vi "RT Main.vi"() -> ()   [LabVIEW 2022 SP3]
uses:
  RT Controls/RT All Notifer.ctl
  RT Controls/Main RT Case.ctl
  RT Sub VI's/RT Global.vi
panel:
  out "Iteration":i32
  out "Status":bool
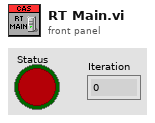
[diagram p1: front panel]
types:
  T1 = enum16{"Init", "Read 'All'", "Read 'n'", "Read '1'", "Write '1'", "Write 'n'", "Write 'All'"}
  T2 = typedef "Main RT Case.ctl" = enum16{"initialize", "Wait For Command", "Wai For Connection"}
  T3 = typedef "RT All Notifer.ctl" = cluster{"Start DAQ":refnum<notifier>, "Sequence":refnum<notifier>}
  T4 = typedef "RT All Queue.ctl" = cluster{"AI\nAO\nDO\nTC\nACC\nStrain":refnum<queue>[], "DI":refnum<queue>}
  T5 = cluster{"Activate Task":cluster{"Analog input":bool, "Analog Output":bool, "Digital input":bool, "Digital output":bool, "Thermocouple":bool, "Strain Gauge":bool, "Accelerometer":bool}, "Start DAQ":bool, "Start Time":timestamp, "DO Names":string[], "AO Names":string[], "AO Default":dbl[], "DO Default":bool[], "Config":cluster{"AO config":cluster{"Channel_Name":string, "Channel_Number":string, "Default_Value":dbl, "Units":string}[], "AI config":cluster{"Channel_Name":string, "Channel_Number":string, "Pre_Scale_min":dbl, "Pre_Scale_max":dbl, "Sensor_min":dbl, "Sensor_max":dbl, "Units":string}[], "DI config":cluster{"Channel_Name":string, "Channel_Number":string, "Default_Value":bool, "DI invert?":bool}[], "DO config":cluster{"Channel_Name":string, "Channel_Number":string, "Default_Value":bool, "DO invert?":bool}[], "TC config":cluster{"Channel_Name":string, "Channel_Number":string, "Pre_Scale_min":dbl, "Pre_Scale_max":dbl, "units":i32, " type":i32}[], "ACC config":cluster{"Channel_Name":string, "Channel_Number":string, "Pre_Scale_min":dbl, "Pre_Scale_max":dbl, "Terminal configuration":i32, "Sensitivity":dbl, "Sensitivity units":i32}[], "SG config":cluster{"Channel_Name":string, "Channel_Number":string, "Pre_Scale_min":dbl, "Pre_Scale_max":dbl}[], "Strain Gauge Settings":cluster{"poisson ratio":dbl, "nominal gage resistance":dbl, "gage factor":dbl}, "Bridge Settings":cluster{"voltage excitation value":dbl, "voltage excitation source":i32, "initial bridge voltage":dbl, "lead wire resistance":dbl, "strain configuration":i32}, "Sample Rate":cluster{"AI Sample Rate":dbl, "AO Sample Rate":dbl, "DI Sample Rate":dbl, "TC Sample Rate":dbl, "DO Sample Rate":dbl, "SG Sample Rate":dbl, "ACC Sample Rate":dbl}}}
  T6 = cluster{"AO":cluster{"CDT":dbl, "Range":dbl, "Component ID":string}[], "DO":cluster{"CDT":dbl, "Position":bool, "Component ID":string}[], "Launch Time":timestamp}
  T7 = cluster{"AO config":cluster{"Channel_Name":string, "Channel_Number":string, "Default_Value":dbl, "Units":string}[], "AI config":cluster{"Channel_Name":string, "Channel_Number":string, "Pre_Scale_min":dbl, "Pre_Scale_max":dbl, "Sensor_min":dbl, "Sensor_max":dbl, "Units":string}[], "DI config":cluster{"Channel_Name":string, "Channel_Number":string, "Default_Value":bool, "DI invert?":bool}[], "DO config":cluster{"Channel_Name":string, "Channel_Number":string, "Default_Value":bool, "DO invert?":bool}[], "TC config":cluster{"Channel_Name":string, "Channel_Number":string, "Pre_Scale_min":dbl, "Pre_Scale_max":dbl, "units":i32, " type":i32}[], "ACC config":cluster{"Channel_Name":string, "Channel_Number":string, "Pre_Scale_min":dbl, "Pre_Scale_max":dbl, "Terminal configuration":i32, "Sensitivity":dbl, "Sensitivity units":i32}[], "SG config":cluster{"Channel_Name":string, "Channel_Number":string, "Pre_Scale_min":dbl, "Pre_Scale_max":dbl}[], "Strain Gauge Settings":cluster{"poisson ratio":dbl, "nominal gage resistance":dbl, "gage factor":dbl}, "Bridge Settings":cluster{"voltage excitation value":dbl, "voltage excitation source":i32, "initial bridge voltage":dbl, "lead wire resistance":dbl, "strain configuration":i32}, "Sample Rate":cluster{"AI Sample Rate":dbl, "AO Sample Rate":dbl, "DI Sample Rate":dbl, "TC Sample Rate":dbl, "DO Sample Rate":dbl, "SG Sample Rate":dbl, "ACC Sample Rate":dbl}}
  T8 = cluster{"Analog input":bool, "Analog Output":bool, "Digital input":bool, "Digital output":bool, "Thermocouple":bool, "Strain Gauge":bool, "Accelerometer":bool}
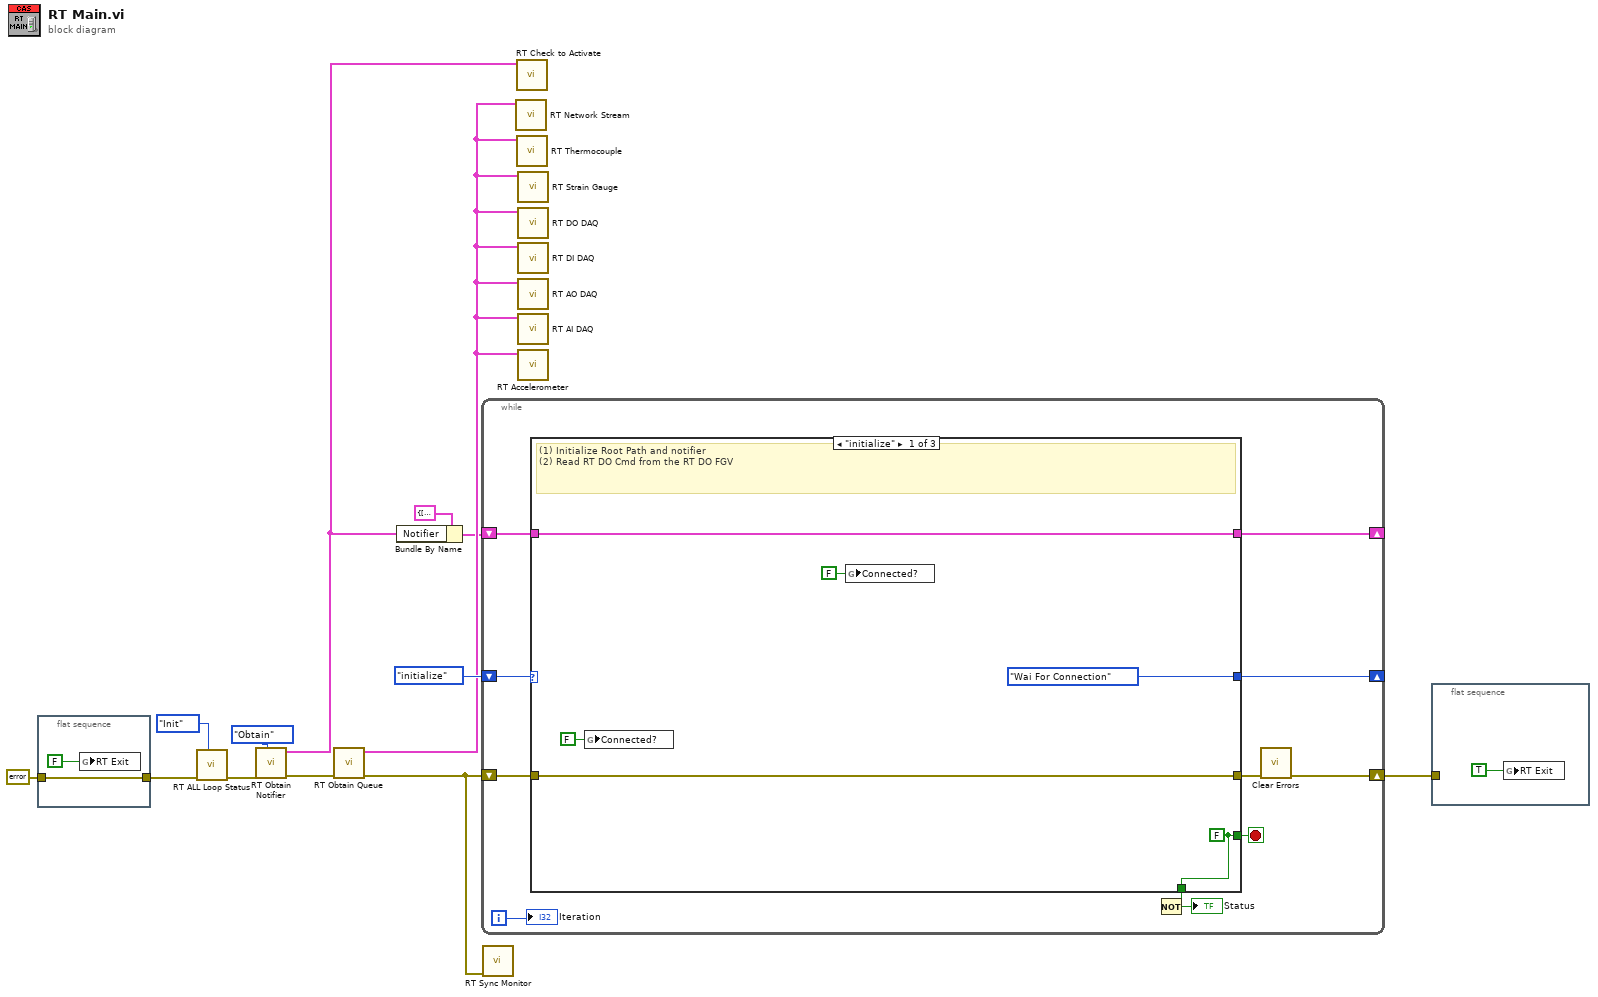
[diagram p0: block diagram]
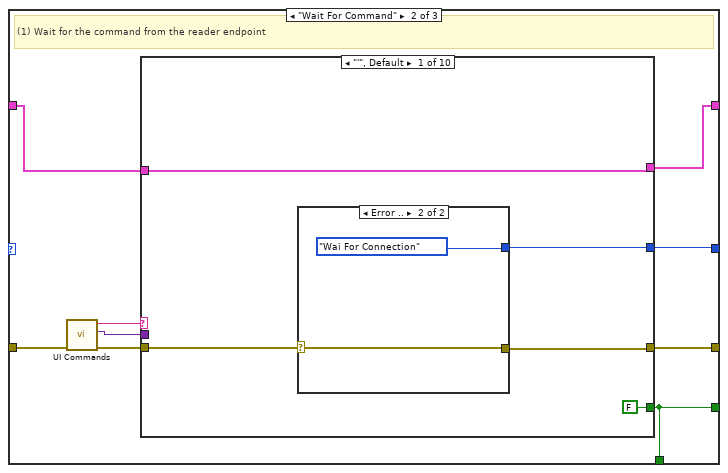
[diagram p2: hidden frame]
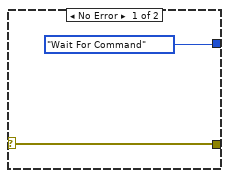
[diagram p3: hidden frame]
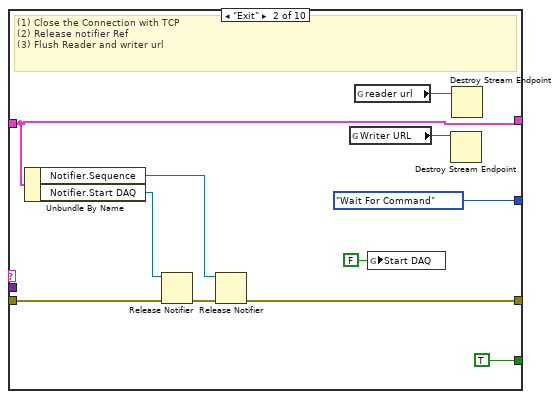
[diagram p4: hidden frame]
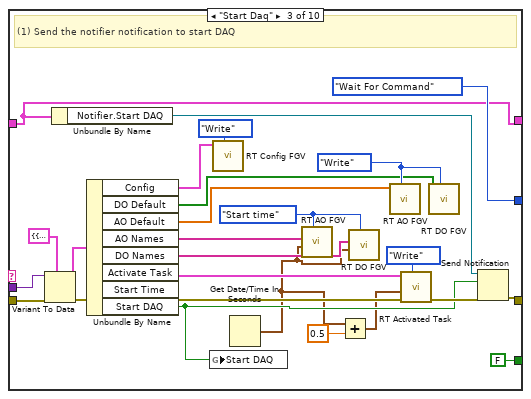
[diagram p5: hidden frame]
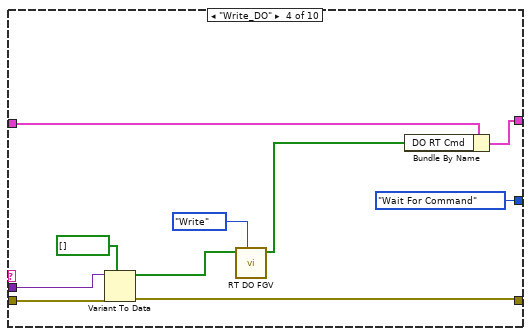
[diagram p6: hidden frame]
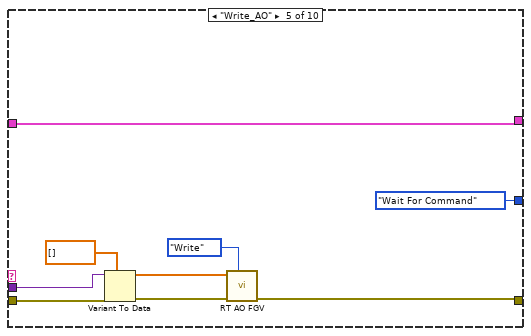
[diagram p7: hidden frame]
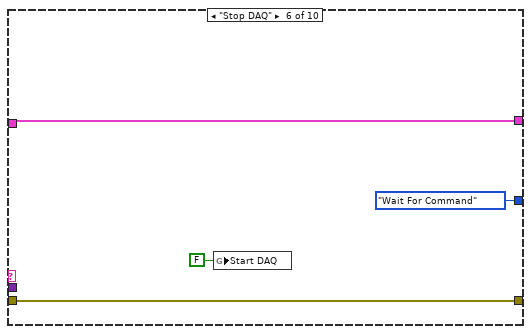
[diagram p8: hidden frame]
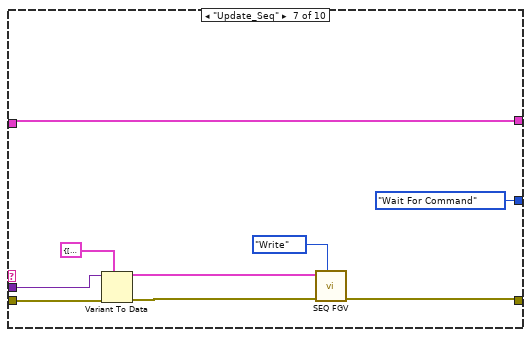
[diagram p9: hidden frame]
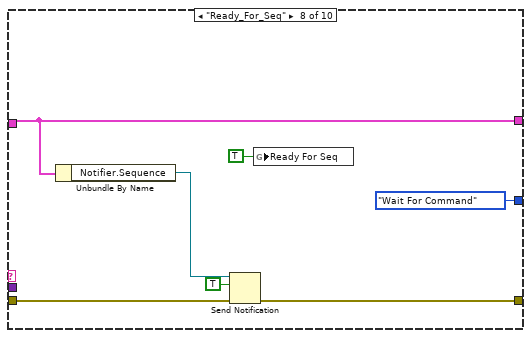
[diagram p10: hidden frame]
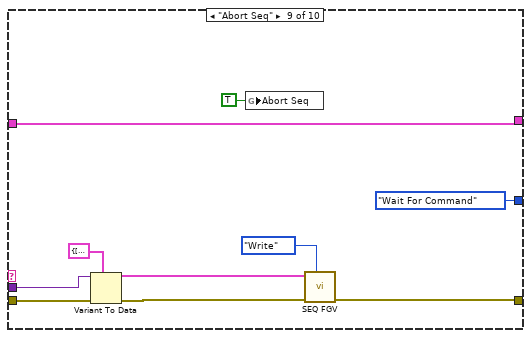
[diagram p11: hidden frame]
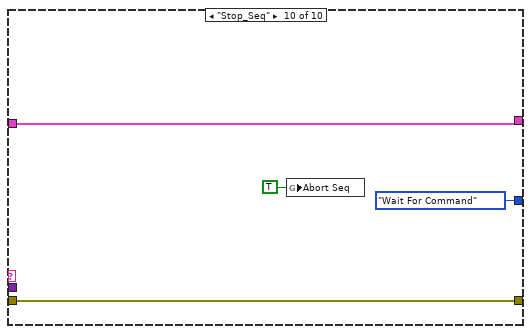
[diagram p12: hidden frame]
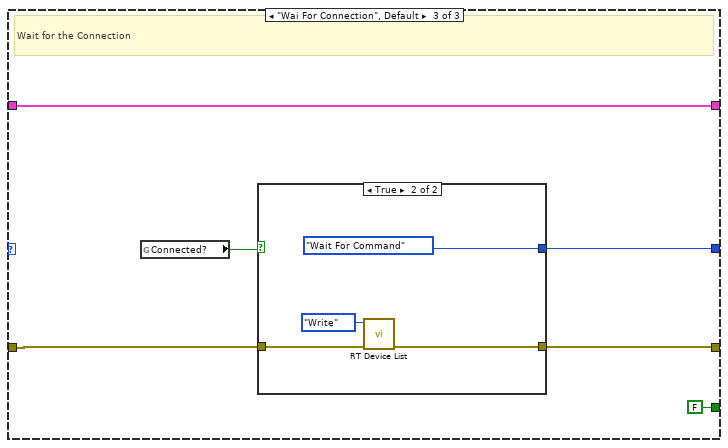
[diagram p13: hidden frame]
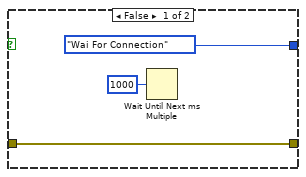
[diagram p14: hidden frame]
diagram:
  n1 = flat-sequence {
    tunnel: errorcluster {"status"=FALSE, "code"=0, "source"=""} ("error in (no error)") -> [w15]
    tunnel: [w15] -> w5
    frame #0 {
      n2 = global write "RT Global.vi" "RT Exit"(FALSE ("Start DAQ")) -> ()
    }
  }
  n3 = call "RT ALL Loop Status.vi"("Option"=T1."Init", "error in (no error)"=w5) -> ("error out"=w4:errorcluster)  [unwired: 7 in, 2 out]
  n4 = call "RT Obtain Notifier.vi"("Case"=enum16{"Obtain", "Read"}."Obtain", "error in (no error)"=w4) -> ("error out"=w8:errorcluster, "All Notifier"=w2:T3)  [unwired: 8 in]
  n5 = call "RT Obtain Queue.vi"("error in"=w8) -> ("error out"=w1:errorcluster, "Queue ref"=w12:T4)  [unwired: 9 in]
  n6 = Bundle By Name(cluster=cluster{"DO RT Cmd":bool[], " Notifier":T3} {"DO RT Cmd"=[], " Notifier"={"Start DAQ"=refnum, "Sequence"=refnum}}, "Notifier"=w2) -> (w6:cluster{"DO RT Cmd":bool[], " Notifier":T3})
  n7 = while {
    shift-right: [w16] -> w11
    shift-left: w1 -> [w25]
    shift-right: [w18] -> _
    shift-left: w6 -> [w17]
    shift-right: [w23] -> _
    shift-left: Main_RT_Case."initialize" -> [w26]
    i -> [w22]
    stop <- w24 stop-if-true
    n8 = case shown="\"initialize\"" w26 {
      tunnel: w25 -> [w32 w36 w140]
      tunnel: [w32 w41 w139] -> w19
      tunnel: [w30 w37 FALSE] -> w24
      tunnel: w17 -> [w31 w40 w144]
      tunnel: [w31 w39 w144] -> w18
      tunnel: [Main_RT_Case."Wai For Connection" w38 w143] -> w23
      tunnel: [w30 w37 _] -> w20
      frame "initialize" {
        w30 = FALSE
        # "(1) Initialize Root Path and notifier\n(2) Read RT DO Cmd from the RT DO FGV"
        n9 = global write "RT Global.vi" "Connected?"(FALSE ("Connected?")) -> ()
        n10 = global write "RT Global.vi" "Connected?"(FALSE ("Connected?")) -> ()
      }
      frame "Wait For Command" {
        # "(1) Wait for the command from the reader endpoint"
        n11 = call "UI Commands.vi"("error in (no error)"=w36) -> ("error out"=w35:errorcluster, "data"=w33:variant, "Message"=w34:string)  [unwired: 8 in]
        n12 = case shown="\"'\", Default" w34 {
          tunnel: [w44 w52 w86 w91 w100 w106 w113 w122 w126 w135] -> w41
          tunnel: [FALSE TRUE FALSE _ _ _ _ _ _ _] -> w37
          tunnel: w40 -> [w46 w56 w81 w95 w104 w108 w110 w121 w134 w138]
          tunnel: [w46 w56 w81 w96 w104 w108 w110 w121 w134 w138] -> w39
          tunnel: [w45 Main_RT_Case."Wait For Command" Main_RT_Case."Wait For Command" Main_RT_Case."Wait For Command" Main_RT_Case."Wait For Command" Main_RT_Case."Wait For Command" Main_RT_Case."Wait For Command" Main_RT_Case."Wait For Command" Main_RT_Case."Wait For Command" Main_RT_Case."Wait For Command"] -> w38
          tunnel: w35 -> [w42 w54 w84 w92 w102 w106 w117 w123 w127 w135]
          tunnel: w33 -> [_ _ w83 w89 w101 _ w116 _ w125 _]
          frame "'", Default {
            n13 = case shown="Error .." w42 {
              selector: w42 -> [w48 w50]
              tunnel: [Main_RT_Case."Wait For Command" Main_RT_Case."Wai For Connection"] -> w45
              tunnel: [w48 w50] -> w44
              frame No Error {
              }
              frame Error {
              }
            }
          }
          frame "Exit" {
            # "(1) Close the Connection with TCP \n(2) Release notifier Ref\n(3) Flush Reader and writer url"
            n14 = Unbundle By Name(w56) -> ("Notifier.Sequence"=w51:refnum<notifier>, "Notifier.Start DAQ"=w55:refnum<notifier>)
            n15 = Release Notifier(notifier=w55, error in (no error)=w54) -> (error out=w53:errorcluster)  [unwired: 1 in, 2 out]
            n16 = Release Notifier(notifier=w51, error in (no error)=w53) -> (error out=w52:errorcluster)  [unwired: 1 in, 2 out]
            n17 = global read "RT Global.vi" "Writer URL"() -> (w60:refnum<k21>)
            n18 = global read "RT Global.vi" "reader url"() -> (w57:refnum<k21>)
            n19 = global write "RT Global.vi" "Start DAQ"(FALSE ("Start DAQ")) -> ()
            n20 = Destroy Stream Endpoint(11:w60) -> ()  [unwired: 1 in, 1 out]
            n21 = Destroy Stream Endpoint(11:w57) -> ()  [unwired: 1 in, 1 out]
          }
          frame "Start Daq" {
            w72 = enum16{"Read", "Write", "Start time", "init"}."Write" ("Enum")
            w73 = enum16{"Read", "Write", "Start time", "init"}."Start time" ("Enum")
            # "(1) Send the notifier notification to start DAQ"
            n22 = Variant To Data(error in=w84, type=T5 {"Activate Task"={"Analog input"=TRUE, "Analog Output"=TRUE, "Digital input"=TRUE, "Digital output"=TRUE, "Thermocouple"=FALSE, "Strain Gauge"=TRUE, "Accelerometer"=TRUE}, "Start DAQ"=TRUE, "Start Time"=timestamp(0 s since 1904-01-01), "DO Names"=[], "AO Names"=[], "AO Default"=[], "DO Default"=[], "Config"={"AO config"=[], "AI config"=[], "DI config"=[], "DO config"=[], "TC config"=[{"Channel_Name"="", "Channel_Number"="", "Pre_Scale_min"=0.0, "Pre_Scale_max"=0.0, "units"=4, " type"=7}], "ACC config"=[], "SG config"=[], "Strain Gauge Settings"={"poisson ratio"=0.3, "nominal gage resistance"=120.0, "gage factor"=2.08}, "Bridge Settings"={"voltage excitation value"=3.3, "voltage excitation source"=10200, "initial bridge voltage"=0.0, "lead wire resistance"=1.7, "strain configuration"=10271}, "Sample Rate"={"AI Sample Rate"=0.0, "AO Sample Rate"=0.0, "DI Sample Rate"=0.0, "TC Sample Rate"=0.0, "DO Sample Rate"=0.0, "SG Sample Rate"=0.0, "ACC Sample Rate"=0.0}}}, Variant=w83) -> (data=w79:T5, error out=w78:errorcluster)
            n23 = Unbundle By Name(w81) -> ("Notifier.Start DAQ"=w80:refnum<notifier>)
            n24 = Unbundle By Name(w79) -> ("Config"=w66:T7, "DO Default"=w68:bool[], "AO Default"=w69:dbl[], "AO Names"=w70:string[], "DO Names"=w71:string[], "Activate Task"=w76:T8, "Start DAQ"=w75:bool)  [unwired: 1 out]
            n25 = global write "RT Global.vi" "Start DAQ"(w75) -> ()
            n26 = call "RT Config FGV.vi"("Enum"=enum16{"Read", "Write"}."Write", "Data"=w66) -> ()  [unwired: 8 in, 2 out]
            n27 = Get Date/Time In Seconds() -> (seconds since 1Jan1904=w64:timestamp)
            n28 = call "RT AO FGV.vi"("Enum"=w73, "Start Time"=w64, "AO Channel Names"=w70) -> ()  [unwired: 6 in, 3 out]
            n29 = Add(x=w64, y=0.5) -> (x+y=w62:timestamp)
            n30 = call "RT DO FGV.vi"("Enum"=w73, "Start Time"=w64, "DO Channel Names"=w71) -> ()  [unwired: 6 in, 3 out]
            n31 = call "RT AO FGV.vi"("Enum"=w72, "AO in"=w69) -> ()  [unwired: 7 in, 3 out]
            n32 = call "RT Activated Task.vi"("Enum"=enum16{"Read", "Write"}."Write", "error in (no error)"=w78, "Start Time in"=w62, "Activate Task"=w76) -> ("error out"=w77:errorcluster)  [unwired: 5 in, 2 out]
            n33 = call "RT DO FGV.vi"("Enum"=w72, "DO in"=w68) -> ()  [unwired: 7 in, 3 out]
            n34 = Send Notification(notification=w75, notifier=w80, error in (no error)=w77) -> (error out=w86:errorcluster)  [unwired: 1 out]
          }
          frame "Write_DO" {
            n35 = Variant To Data(error in=w92, type=bool[] [] ("DO RT Cmd"), Variant=w89) -> (data=w93:bool[], error out=w91:errorcluster)
            n36 = call "RT DO FGV.vi"("Enum"=enum16{"Read", "Write", "Start time", "init"}."Write", "DO in"=w93) -> ("DO out"=w87:bool[])  [unwired: 7 in, 2 out]
            n37 = Bundle By Name(cluster=w95, "DO RT Cmd"=w87) -> (w96:cluster{"DO RT Cmd":bool[], " Notifier":T3})
          }
          frame "Write_AO" {
            n38 = Variant To Data(error in=w102, type=dbl[] [], Variant=w101) -> (data=w98:dbl[], error out=w100:errorcluster)
            n39 = call "RT AO FGV.vi"("Enum"=enum16{"Read", "Write", "Start time", "init"}."Write", "AO in"=w98) -> ()  [unwired: 7 in, 3 out]
          }
          frame "Stop DAQ" {
            n40 = global write "RT Global.vi" "Start DAQ"(FALSE ("Start DAQ")) -> ()
          }
          frame "Update_Seq" {
            n41 = Variant To Data(error in=w117, type=T6 {"AO"=[], "DO"=[], "Launch Time"=timestamp(0 s since 1904-01-01)}, Variant=w116) -> (data=w114:T6, error out=w115:errorcluster)
            n42 = call "SEQ FGV.vi"("Enum"=enum16{"Read", "Write"}."Write", "error in (no error)"=w115, "Seq data in"=w114) -> ("error out"=w113:errorcluster)  [unwired: 7 in, 1 out]
          }
          frame "Ready_For_Seq" {
            n43 = Unbundle By Name(w121) -> ("Notifier.Sequence"=w120:refnum<notifier>)
            n44 = Send Notification(notification=TRUE, notifier=w120, error in (no error)=w123) -> (error out=w122:errorcluster)  [unwired: 1 out]
            n45 = global write "RT Global.vi" "Ready For Seq"(TRUE ("RT Exit")) -> ()
          }
          frame "Abort Seq" {
            n46 = Variant To Data(error in=w127, type=T6 {"AO"=[], "DO"=[], "Launch Time"=timestamp(0 s since 1904-01-01)}, Variant=w125) -> (data=w129:T6, error out=w130:errorcluster)
            n47 = global write "RT Global.vi" "Abort Seq"(TRUE ("Abort Seq")) -> ()
            n48 = call "SEQ FGV.vi"("Enum"=enum16{"Read", "Write"}."Write", "error in (no error)"=w130, "Seq data in"=w129) -> ("error out"=w126:errorcluster)  [unwired: 7 in, 1 out]
          }
          frame "Stop_Seq" {
            n49 = global write "RT Global.vi" "Abort Seq"(TRUE ("Abort Seq")) -> ()
          }
        }
      }
      frame "Wai For Connection", Default {
        # "Wait for the Connection"
        n50 = global read "RT Global.vi" "Connected?"() -> (w141:bool)
        n51 = case shown="True" w141 {
          tunnel: [Main_RT_Case."Wai For Connection" Main_RT_Case."Wait For Command"] -> w143
          tunnel: w140 -> [w145 w149]
          tunnel: [w145 w148] -> w139
          frame False {
            n52 = Wait Until Next ms Multiple(millisecond multiple=u32 1000 ("milliseconds to wait")) -> ()  [unwired: 1 out]
          }
          frame True {
            n53 = call "RT Device List.vi"("error in (no error)"=w149, "Enum"=enum16{"Read", "Write"}."Write") -> ("error out"=w148:errorcluster)  [unwired: 7 in, 1 out]
          }
        }
      }
    }
    n54 = Not(x=w20) -> (.not. x?=→"Status":bool)
    n55 = call <vilib>:"Clear Errors.vi"("error in (no error)"=w19) -> ("error out"=w16:errorcluster)  [unwired: 5 in, 1 out]
    "Iteration" <- w22
  }
  n56 = call "RT Sync Monitor.vi"("error in (no error)"=w1) -> ()  [unwired: 10 in, 1 out]
  n57 = call "RT Network Stream.vi"("Queue ref"=w12) -> ()  [unwired: 11 in]
  n58 = call "RT Check to Activate.vi"("All Notifier"=w2) -> ()  [unwired: 11 in]
  n59 = call "RT Thermocouple.vi"("Queue ref"=w12) -> ()  [unwired: 11 in]
  n60 = call "RT Strain Gauge.vi"("Queue ref"=w12) -> ()  [unwired: 11 in]
  n61 = call "RT DO DAQ.vi"("Queue ref"=w12) -> ()  [unwired: 11 in]
  n62 = call "RT DI DAQ.vi"("Queue ref"=w12) -> ()  [unwired: 11 in]
  n63 = call "RT AO DAQ.vi"("Queue ref"=w12) -> ()  [unwired: 11 in]
  n64 = call "RT AI DAQ.vi"("Queue ref"=w12) -> ()  [unwired: 11 in]
  n65 = call "RT Accelerometer.vi"("Queue ref"=w12) -> ()  [unwired: 11 in]
  n66 = flat-sequence {
    tunnel: w11 -> [_]
    frame #0 {
      n67 = global write "RT Global.vi" "RT Exit"(TRUE ("Start DAQ")) -> ()
    }
  }
